vi "test_DependencyList_subCheckPathAndName.vi"() -> (3 "Pass?":bool)   [LabVIEW 2020, in "Tests.DependencyInspection.lvlib"]
uses:
  Tests.DependencyInspection.lvlib
  Validation/Input_PathInfo.ctl
  Validation/Validate_CheckPathAndName.ctl
  CDependencyList/CDependencyList.lvclass
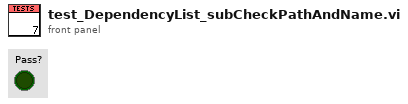
[diagram p1: front panel]
types:
  T1 = typedef "Tests.DependencyInspection.lvlib/Validate_CheckPathAndName.ctl" = cluster{"path to check?":bool, "path out":path}
  T2 = typedef "Tests.DependencyInspection.lvlib/Input_PathInfo.ctl" = cluster{"path":path, "delimited name":string, "parent path":path, "exclude instances?":bool}
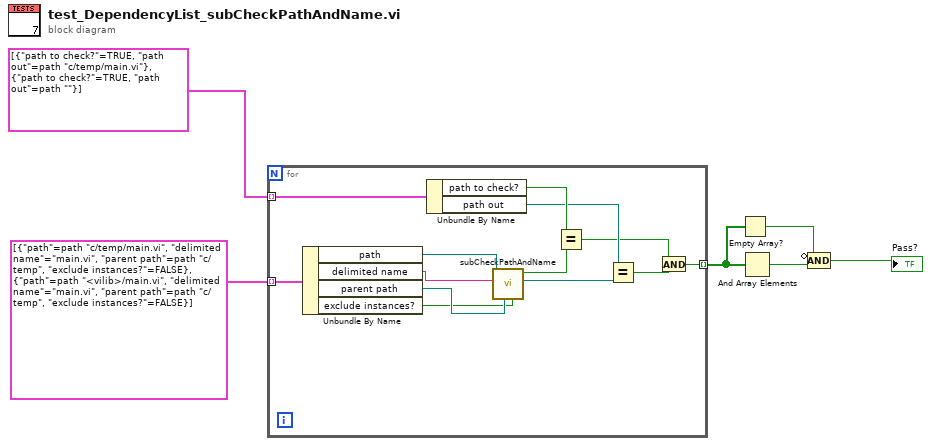
[diagram p0: block diagram]
diagram:
  n1 = for {
    tunnel: T2[] [{"path"=path "c:/temp/main.vi", "delimited name"="main.vi", "parent path"=path "c:/temp", "exclude instances?"=FALSE}, {"path"=path "<vilib>/main.vi", "delimited name"="main.vi", "parent path"=path "c:/temp", "exclude instances?"=FALSE}] -> [w19] mode=indexing
    tunnel: T1[] [{"path to check?"=TRUE, "path out"=path "c:/temp/main.vi"}, {"path to check?"=TRUE, "path out"=path ""}] -> [w14] mode=indexing
    tunnel: [w7] -> w4 mode=indexing
    n2 = Unbundle By Name(w19) -> ("path"=w18:path, "delimited name"=w17:string, "parent path"=w16:path, "exclude instances?"=w15:bool)
    n3 = Unbundle By Name(w14) -> ("path to check?"=w13:bool, "path out"=w11:path)
    n4 = call "subCheckPathAndName.vi"("exclude instances?"=w15, "parent path"=w16, "delimited name"=w17, "path"=w18) -> ("path out"=w10:path, "path to check?"=w12:bool)  [unwired: 6 in]
    n5 = Equal?(x=w13, y=w12) -> (x = y?=w9:bool)
    n6 = Equal?(x=w11, y=w10) -> (x = y?=w8:bool)
    n7 = And(x=w9, y=w8) -> (x .and. y?=w7:bool)
  }
  n8 = Empty Array?(array=w4) -> (empty?=w2:bool)
  n9 = And Array Elements(Boolean array=w4) -> (logical AND=w3:bool)
  n10 = Compound Arithmetic op=AND(invert w2, w3) -> (→"Pass?":bool)
